vi "Config Panel_2.vi"() -> ()   [LabVIEW 2018]
panel:
  in  "Restore Default ch1 4":bool
  in  "Copy to Input ch1 4":bool
  in  "Set from Input ch1 4":bool
  in  "Restore Default ch1 3":bool
  in  "Copy to Input ch1 3":bool
  in  "Set from Input ch1 3":bool
  in  "Restore Default ch1 2":bool
  in  "Copy to Input ch1 2":bool
  in  "Set from Input ch1 2":bool
  in  "Restore Default ch1":bool
  in  "Copy to Input ch1":bool
  in  "Set from Input ch1":bool
  in  "Cancel Button":bool
  in  "Copy Button":bool
  in  "Restore Button":bool
  in  "Set from Input Button":bool
  in  "Load Default Button":bool
  in  "Close Button":bool
  out "Current Configuration File:":string
  in  "Input Cluster":T1={"Parameters"={"Image\nInitial Line"=0.0, "Image\nInitial Column"=0.0, "Image\nFinal Line"=0.0, "Image\nFInal Column"=0.0, "Vertical\nBinning"=0.0, "Horizontal\nBinning"=0.0, "Pre-amplification\nGain"=0.0, "CCD\nEM Gain"=0.0, "Output\nAmplifier Mode"="", "Readout\nRate"=0.0, "Shutter\nOpenning Time"=0.0, "Shutter\nClosing Time"=0.0, "Vertical\nShift Speed"=0.0, "Read\nMode"=0.0, "Vertical\nClock Voltage"=0.0, "A/D Converter\nNumber"=0.0, "Shutter\nMode"="Open", "Shutter\nSignal Level"="High", "Trigger\nMode"="Internal", "Frame\nTransfer"="On", "Acquisition\nMode"="Kinetic"}}
  in  "Save As Button":bool
  in  "Save Button":bool
  in  "Load Button":bool
  in  "Radio Buttons":T2(radio)
  in  "Scrollbar":i32(c297)
  out "Cameras Cluster":T3={"Current Configuration"={"Image\nInitial Line"=0.0, "Image\nInitial Column"=0.0, "Image\nFinal Line"=0.0, "Image\nFInal Column"=0.0, "Vertical\nBinning"=0.0, "Horizontal\nBinning"=0.0, "Pre-amplification\nGain"=0.0, "CCD\nEM Gain"=0.0, "Readout\nRate"=0.0, "Shutter\nOpenning Time"=0.0, "Shutter\nClosing Time"=0.0, "Vertical\nShift Speed"=0.0, "Read\nMode"=0.0, "Vertical\nClock Voltage"=0.0, "A/D Converter\nNumber"=0.0, "Image\nInitial Line 2"=0.0, "Image\nInitial Column 2"=0.0, "Image\nFinal Line 2"=0.0, "Image\nFInal Column 2"=0.0, "Vertical\nBinning 2"=0.0, "Horizontal\nBinning 2"=0.0, "Pre-amplification\nGain 2"=0.0, "CCD\nEM Gain 2"=0.0, "Readout\nRate 2"=0.0, "Shutter\nOpenning Time 2"=0.0, "Shutter\nClosing Time 2"=0.0, "Vertical\nShift Speed 2"=0.0, "Read\nMode 2"=0.0, "Vertical\nClock Voltage 2"=0.0, "A/D Converter\nNumber 2"=0.0, "Image\nInitial Line 3"=0.0, "Image\nInitial Column 3"=0.0, "Image\nFinal Line 3"=0.0, "Image\nFInal Column 3"=0.0, "Vertical\nBinning 3"=0.0, "Horizontal\nBinning 3"=0.0, "Pre-amplification\nGain 3"=0.0, "CCD\nEM Gain 3"=0.0, "Readout\nRate 3"=0.0, "Shutter\nOpenning Time 3"=0.0, "Shutter\nClosing Time 3"=0.0, "Vertical\nShift Speed 3"=0.0, "Read\nMode 3"=0.0, "Vertical\nClock Voltage 3"=0.0, "A/D Converter\nNumber 3"=0.0, "Image\nInitial Line 4"=0.0, "Image\nInitial Column 4"=0.0, "Image\nFinal Line 4"=0.0, "Image\nFInal Column 4"=0.0, "Vertical\nBinning 4"=0.0, "Horizontal\nBinning 4"=0.0, "Pre-amplification\nGain 4"=0.0, "CCD\nEM Gain 4"=0.0, "Readout\nRate 4"=0.0, "Shutter\nOpenning Time 4"=0.0, "Shutter\nClosing Time 4"=0.0, "Vertical\nShift Speed 4"=0.0, "Read\nMode 4"=0.0, "Vertical\nClock Voltage 4"=0.0, "A/D Converter\nNumber 4"=0.0, "Shutter\nMode 3"="Open", "Shutter\nMode 4"="Open", "Shutter\nMode 5"="Open", "Shutter\nMode 6"="Open", "Shutter\nSignal Level"="High", "Shutter\nSignal Level 2"="High", "Shutter\nSignal Level 3"="High", "Shutter\nSignal Level 4"="High", "Trigger\nMode"="Internal", "Trigger\nMode 2"="Internal", "Trigger\nMode 3"="Internal", "Trigger\nMode 4"="Internal", "Frame\nTransfer"="On", "Frame\nTransfer 2"="On", "Frame\nTransfer 3"="On", "Frame\nTransfer 4"="On", "Acquisition\nMode"="Kinetic", "Acquisition\nMode 2"="Kinetic", "Acquisition\nMode 3"="Kinetic", "Acquisition\nMode 4"="Kinetic", "Output\nAmplifier Mode"="", "Output\nAmplifier Mode 2"="", "Output\nAmplifier Mode 3"="", "Output\nAmplifier Mode 4"=""}}
  # "Current Configuration Parameters\nChannel 1          Channel 2          Channel 3          Channel 4"
  # "Parameter Input"
  # "Selected Channel \nOperations:"
  # "Operations:"
  # "File Operations:\n(apply for all channels)"
  # "NOTAS:\n\"Current Configuration:\" seria: \"ic_sparc_default.cfg\" ou \"ic_sparc.cfg\" ou o nome utilizado pelo usuário em \"Save As\".  \nO botão \"Close Configuration Panel\" representa a forma apropriada para fechar o painel de configuração dentro do S4GUI."
  # "Channel Selection:"
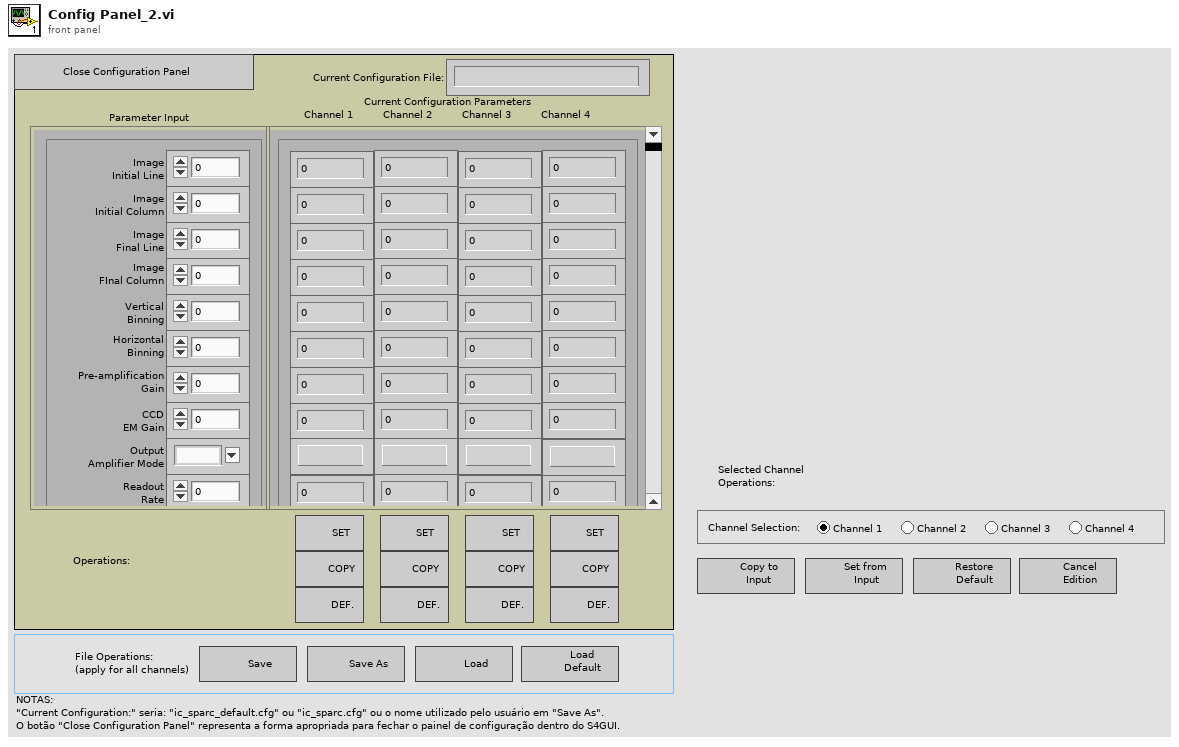
[diagram p1: front panel]
types:
  T1 = cluster{"Parameters":cluster{"Image\nInitial Line":dbl, "Image\nInitial Column":dbl, "Image\nFinal Line":dbl, "Image\nFInal Column":dbl, "Vertical\nBinning":dbl, "Horizontal\nBinning":dbl, "Pre-amplification\nGain":dbl, "CCD\nEM Gain":dbl, "Output\nAmplifier Mode":string, "Readout\nRate":dbl, "Shutter\nOpenning Time":dbl, "Shutter\nClosing Time":dbl, "Vertical\nShift Speed":dbl, "Read\nMode":dbl, "Vertical\nClock Voltage":dbl, "A/D Converter\nNumber":dbl, "Shutter\nMode":string, "Shutter\nSignal Level":string, "Trigger\nMode":string, "Frame\nTransfer":string, "Acquisition\nMode":string}}
  T2 = enum32{"Radio Selection 1", "Radio Selection 2", "Radio Selection 3", "Radio Selection 4"}
  T3 = cluster{"Current Configuration":cluster{"Image\nInitial Line":dbl, "Image\nInitial Column":dbl, "Image\nFinal Line":dbl, "Image\nFInal Column":dbl, "Vertical\nBinning":dbl, "Horizontal\nBinning":dbl, "Pre-amplification\nGain":dbl, "CCD\nEM Gain":dbl, "Readout\nRate":dbl, "Shutter\nOpenning Time":dbl, "Shutter\nClosing Time":dbl, "Vertical\nShift Speed":dbl, "Read\nMode":dbl, "Vertical\nClock Voltage":dbl, "A/D Converter\nNumber":dbl, "Image\nInitial Line 2":dbl, "Image\nInitial Column 2":dbl, "Image\nFinal Line 2":dbl, "Image\nFInal Column 2":dbl, "Vertical\nBinning 2":dbl, "Horizontal\nBinning 2":dbl, "Pre-amplification\nGain 2":dbl, "CCD\nEM Gain 2":dbl, "Readout\nRate 2":dbl, "Shutter\nOpenning Time 2":dbl, "Shutter\nClosing Time 2":dbl, "Vertical\nShift Speed 2":dbl, "Read\nMode 2":dbl, "Vertical\nClock Voltage 2":dbl, "A/D Converter\nNumber 2":dbl, "Image\nInitial Line 3":dbl, "Image\nInitial Column 3":dbl, "Image\nFinal Line 3":dbl, "Image\nFInal Column 3":dbl, "Vertical\nBinning 3":dbl, "Horizontal\nBinning 3":dbl, "Pre-amplification\nGain 3":dbl, "CCD\nEM Gain 3":dbl, "Readout\nRate 3":dbl, "Shutter\nOpenning Time 3":dbl, "Shutter\nClosing Time 3":dbl, "Vertical\nShift Speed 3":dbl, "Read\nMode 3":dbl, "Vertical\nClock Voltage 3":dbl, "A/D Converter\nNumber 3":dbl, "Image\nInitial Line 4":dbl, "Image\nInitial Column 4":dbl, "Image\nFinal Line 4":dbl, "Image\nFInal Column 4":dbl, "Vertical\nBinning 4":dbl, "Horizontal\nBinning 4":dbl, "Pre-amplification\nGain 4":dbl, "CCD\nEM Gain 4":dbl, "Readout\nRate 4":dbl, "Shutter\nOpenning Time 4":dbl, "Shutter\nClosing Time 4":dbl, "Vertical\nShift Speed 4":dbl, "Read\nMode 4":dbl, "Vertical\nClock Voltage 4":dbl, "A/D Converter\nNumber 4":dbl, "Shutter\nMode 3":string, "Shutter\nMode 4":string, "Shutter\nMode 5":string, "Shutter\nMode 6":string, "Shutter\nSignal Level":string, "Shutter\nSignal Level 2":string, "Shutter\nSignal Level 3":string, "Shutter\nSignal Level 4":string, "Trigger\nMode":string, "Trigger\nMode 2":string, "Trigger\nMode 3":string, "Trigger\nMode 4":string, "Frame\nTransfer":string, "Frame\nTransfer 2":string, "Frame\nTransfer 3":string, "Frame\nTransfer 4":string, "Acquisition\nMode":string, "Acquisition\nMode 2":string, "Acquisition\nMode 3":string, "Acquisition\nMode 4":string, "Output\nAmplifier Mode":string, "Output\nAmplifier Mode 2":string, "Output\nAmplifier Mode 3":string, "Output\nAmplifier Mode 4":string}}
  T4 = cluster{"Parameters":refnum<vi>, "Current Configuration":refnum<vi>}
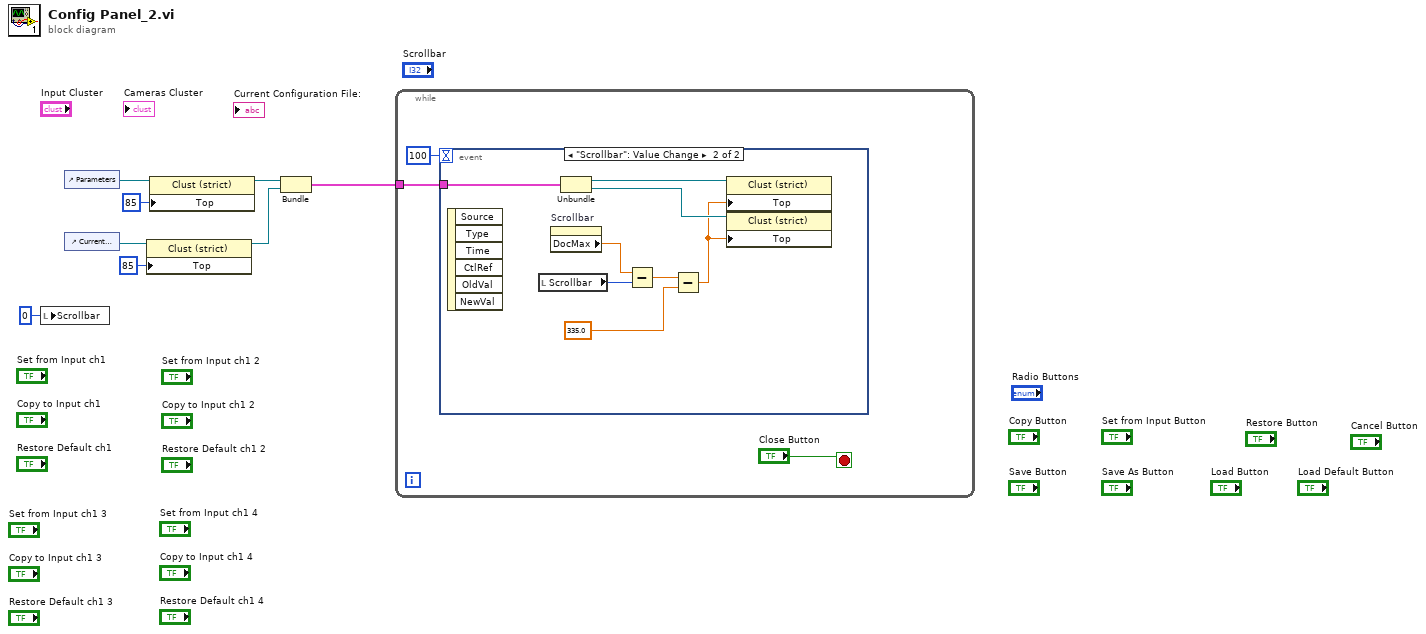
[diagram p0: block diagram]
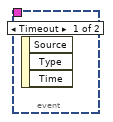
[diagram p2: hidden frame]
diagram:
  n1 = local write "Scrollbar"(0 ("Scrollbar")) -> ()
  n2 = control-ref of="Parameters"() -> (w8:refnum<vi>)
  n3 = control-ref of="Current Configuration"() -> (w7:refnum<vi>)
  n4 = property on="Property Node" class="Clust (strict)"(reference=w7, "Top"=85 ("Position:Top")) -> (reference out=w3:refnum<vi>)  [unwired: 1 in, 1 out]
  n5 = property on="Property Node" class="Clust (strict)"(reference=w8, "Top"=85 ("Position:Top")) -> (reference out=w4:refnum<vi>)  [unwired: 1 in, 1 out]
  n6 = Bundle("Parameters"=w4, "Current Configuration"=w3) -> (w2:T4)  [unwired: 1 in]
  n7 = while {
    tunnel: w2 -> [w10]
    stop <- "Close Button" stop-if-true
    n8 = event shown="[1] \"Scrollbar\": Value Change" {
      selector: _ -> [_ _]
      dyn-events: _ -> [_ _]
      timeout: 100 -> [_ _]
      tunnel: w10 -> [_ w16]
      event Timeout {
        n9 = event-data() -> ()  [unwired: 1 in, 3 out]
      }
      event "Scrollbar": Value Change {
        n10 = event-data() -> ()  [unwired: 1 in, 6 out]
        n11 = local read "Scrollbar"() -> (w19:i32)
        n12 = property on="Scrollbar" class="Scroll (strict)"() -> ("DocMax"=w12:dbl)  [unwired: 2 in, 2 out]
        n13 = Unbundle(w16) -> ("Parameters"=w15:refnum<vi>, "Current Configuration"=w14:refnum<vi>)
        n14 = Subtract(x=w12, y=w19) -> (x-y=w18:dbl)
        n15 = Subtract(x=w18, y=335.0 ("BarOffset")) -> (x-y=w13:dbl)
        n16 = property on="Property Node" class="Clust (strict)"(reference=w15, "Top"=w13) -> ()  [unwired: 1 in, 2 out]
        n17 = property on="Property Node" class="Clust (strict)"(reference=w14, "Top"=w13) -> ()  [unwired: 1 in, 2 out]
      }
    }
  }
